vi "set_ra_table.vi"(8 "error in (no error)":errorcluster, 10 "RAPS points cluster in":T1, 11 "FPGAWrapperMH120124RAPS_PXI7813R in":refnum<class "FPGAWrapperMH120124RAPS_PXI7813R.lvclass">) -> (0 "error out":errorcluster, 3 "FPGAWrapperMH120124RAPS_PXI7813R out":refnum<class "FPGAWrapperMH120124RAPS_PXI7813R.lvclass">)   [LabVIEW 2010, in "FPGAWrapperMH120124RAPS_PXI7813R.lvclass"]
uses:
  FPGAWrapperMH120124RAPS_PXI7813R.lvclass
  Trajectory/TrajectoryMH100122AODRAPS/TrajectoryMH100122AODRAPS/raps_points_cluster.ctl
  FPGAWrapperMH120124RAPS_PXI7813R.lvclass/FPGAWrapperMH120124RAPS_PXI7813R.ctl
  Trajectory/TrajectoryMH100122AODRAPS/TrajectoryMH100122AODRAPS/TrajectoryMH100122AODRAPS.lvclass
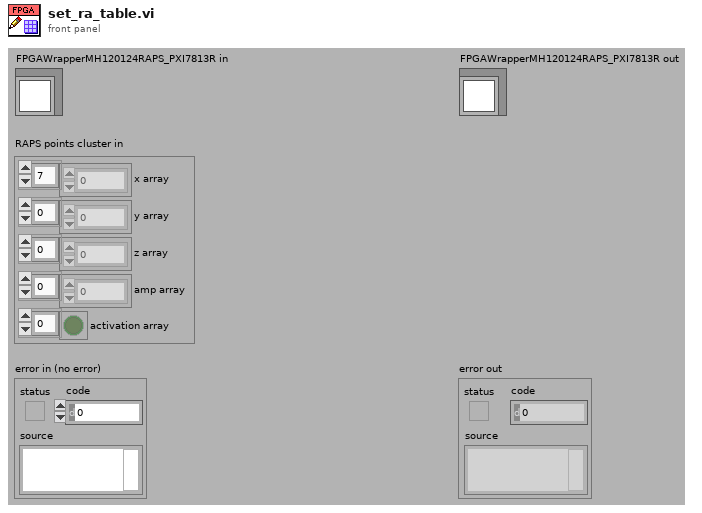
[diagram p1: front panel]
types:
  T1 = typedef "TrajectoryMH100122AODRAPS.lvclass/raps_points_cluster.ctl" = cluster{"x array":u16[], "y array":u16[], "z array":u16[], "amp array":u16[], "activation array":bool[]}
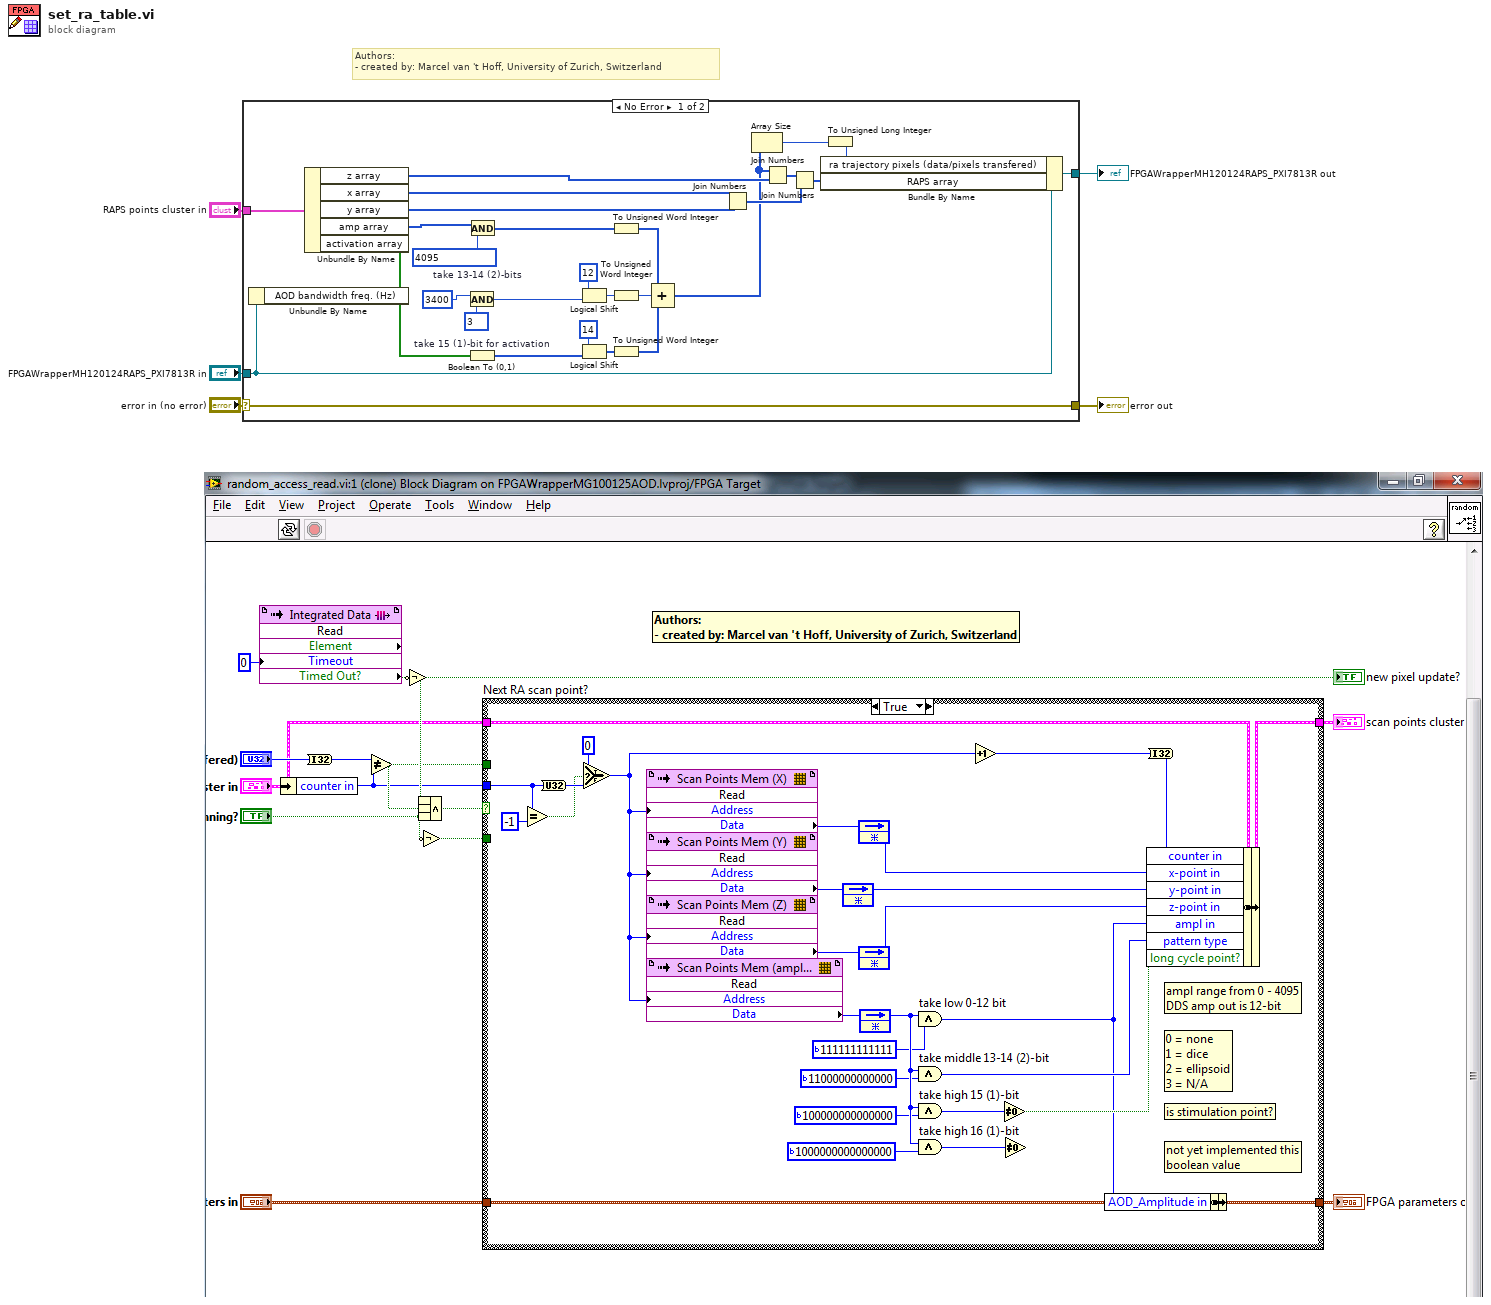
[diagram p0: block diagram]
diagram:
  # "Authors: \n- created by: Marcel van 't Hoff, University of Zurich, Switzerland"
  n1 = case shown="No Error" "error in (no error)" {
    selector: "error in (no error)" -> [w33 w35]
    tunnel: [w33 w35] -> w4
    tunnel: [w14 w34] -> w2
    tunnel: "FPGAWrapperMH120124RAPS_PXI7813R in" -> [w15 w34]
    tunnel: "RAPS points cluster in" -> [w32 _]
    frame No Error {
      n2 = Unbundle By Name(w15) -> ()  [unwired: 1 out]
      n3 = Unbundle By Name(w32) -> ("z array"=w7:u16[], "x array"=w9:u16[], "y array"=w8:u16[], "amp array"=w30:u16[], "activation array"=w13:bool[])
      n4 = And "take 13-14 (2)-bits"(x=u16 3400 ("settings cluster.AOD amplitude"), y=i8 3) -> (x .and. y?=w27:u16)
      n5 = Boolean To (0,1) "take 15 (1)-bit for activation"(Boolean=w13) -> (0, 1=w24:i16[])
      n6 = And(x=w30, y=u16 4095) -> (x .and. y?=w28:u16[])
      n7 = Logical Shift(y=i8 12, x=w27) -> (x << y=w25:u16)
      n8 = Logical Shift(y=i8 14, x=w24) -> (x << y=w22:i16[])
      n9 = To Unsigned Word Integer(number=w28) -> (unsigned 16bit integer=w21:u16[])
      n10 = To Unsigned Word Integer(number=w25) -> (unsigned 16bit integer=w20:u16)
      n11 = To Unsigned Word Integer(number=w22) -> (unsigned 16bit integer=w19:u16[])
      n12 = Compound Arithmetic op=ADD(w21, w20, w19) -> (w6:u16[])
      n13 = Join Numbers(hi=w9, lo=w8) -> ((hi.lo)=w17:u32[])
      n14 = Array Size(array=w6) -> (size(s)=w12:i32)
      n15 = Join Numbers(hi=w6, lo=w7) -> ((hi.lo)=w18:u32[])
      n16 = Join Numbers(hi=w18, lo=w17) -> ((hi.lo)=w16:u64[])
      n17 = To Unsigned Long Integer(number=w12) -> (unsigned 32bit integer=w11:u32)
      n18 = Bundle By Name(cluster=w15, "ra trajectory pixels (data/pixels transfered)"=w11, "RAPS array"=w16) -> (w14:refnum<class "FPGAWrapperMH120124RAPS_PXI7813R.lvclass">)
    }
    frame Error {
    }
  }
  "error out" <- w4
  "FPGAWrapperMH120124RAPS_PXI7813R out" <- w2
